vi "ExSubNPCreateFileStrip.vi"(2 "error in (no error)":errorcluster, 3 "File and Display Name":string, 4 "Camera Handle":u32) -> (0 "error out":errorcluster, 1 "Handles Out":T1)   [LabVIEW 2010]
panel:
  # "ExSubCreateFileStrip:\nThis Sub-VI creates a file and opens it"
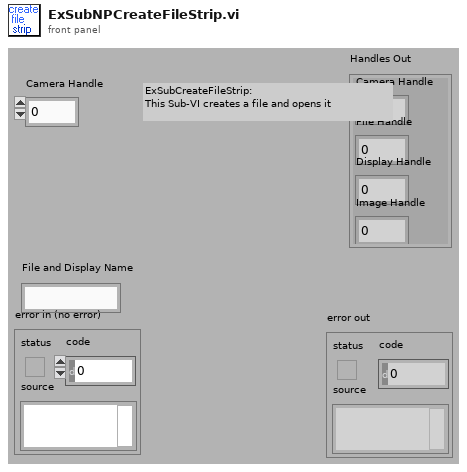
[diagram p1: front panel]
types:
  T1 = cluster{"Camera Handle":u32, "File Handle":u32, "Display Handle":u32, "Image Handle":u32}
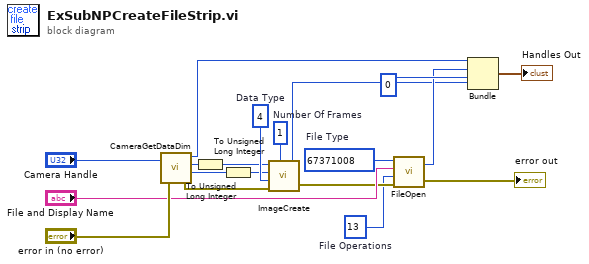
[diagram p0: block diagram]
diagram:
  w8 = 13  # File Operations
  w9 = 67371008  # File Type
  w10 = u32 4  # Data Type
  w11 = u32 1  # Number Of Frames
  n1 = call <userlib>:"CameraGetDataDim.vi"("Camera Handle"="Camera Handle", "error in"="error in (no error)") -> ("Camera Handle"=w4:u32, "Xdim"=w17:u32, "Ydim"=w18:u32, "error out"=w19:errorcluster)
  n2 = To Unsigned Long Integer(number=w17) -> (unsigned 32bit integer=w7:u32)
  n3 = To Unsigned Long Integer(number=w18) -> (unsigned 32bit integer=w6:u32)
  n4 = call <userlib>:"ImageCreate.vi"("X dimension"=w7, "Y dimension"=w6, "Data Type"=w10, "error in"=w19, "Number Of Frames"=w11) -> ("Image Handle"=w1:u32, "error out"=w12:errorcluster)
  n5 = call <userlib>:"FileOpen.vi"("error in"=w12, "File Operations"=w8, "FileName"="File and Display Name", "File Type"=w9) -> ("error out"=→"error out":errorcluster, "File Handle"=w2:u32)
  n6 = Bundle("Camera Handle"=w4, "File Handle"=w2, "Display Handle"=u32 0, "Image Handle"=w1) -> (→"Handles Out":T1)  [unwired: 1 in]
